vi "data_process_packet.vi"(8 "error in (no error)":errorcluster, 10 "T_offset":u32, 11 "Data Packet":string) -> (0 "error out":errorcluster, 1 "Sensor Packets Returned":i32, 2 "Sensor Readings (Signed)":i16[](array[numeric]), 3 "Time":u32)   [LabVIEW 2018]
panel:
  out "Time Packet":string
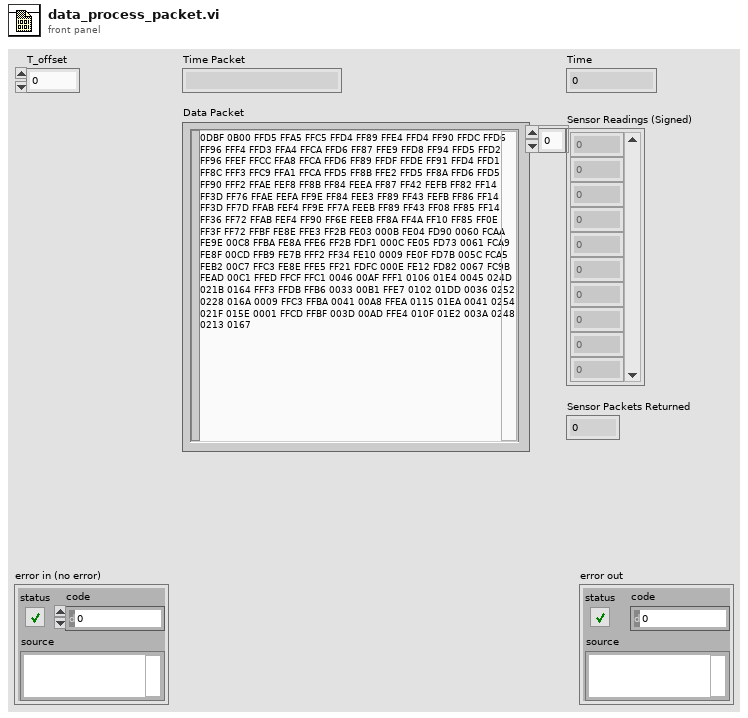
[diagram p1: front panel]
types:
  T1 = enum16{"big-endian, network order", "native, host order", "little-endian"}
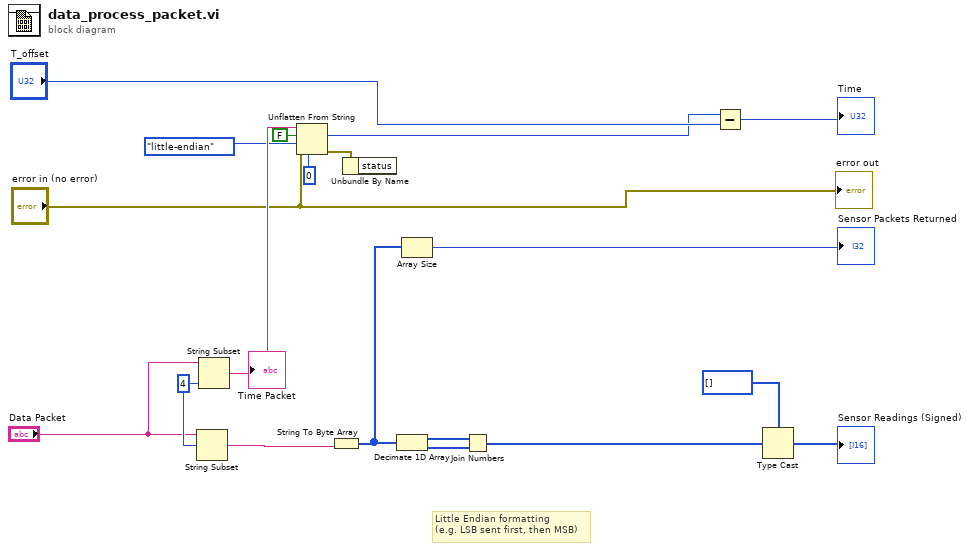
[diagram p0: block diagram]
diagram:
  w19 = 4 ("length (rest)")
  # "Little Endian formatting\n(e.g. LSB sent first, then MSB)"
  n1 = String Subset(string="Data Packet", offset (0)=w19) -> (substring=w16:string)  [unwired: 1 in]
  n2 = String Subset(string="Data Packet", length (rest)=w19) -> (substring=w18:string)  [unwired: 1 in]
  "Time Packet" <- w18
  n3 = Unflatten From String(type=u32 0 ("default (0 U32)"), binary string=w18, data includes array or string size? (T)=FALSE, byte order (0:big-endian, network order)=T1."little-endian", error in (no error)="error in (no error)") -> (value=w2:u32, error out=w4:errorcluster)  [unwired: 1 out]
  n4 = String To Byte Array(string=w16) -> (unsigned byte array=w15:u8[])
  n5 = Unbundle By Name(w4) -> ()  [unwired: 1 out]
  n6 = Decimate 1D Array(w15) -> (w12:u8[], w11:u8[])
  n7 = Array Size(array=w15) -> (size(s)=→"Sensor Packets Returned":i32)
  n8 = Join Numbers(hi=w12, lo=w11) -> ((hi.lo)=w9:u16[])
  n9 = Subtract(x=w2, y="T_offset") -> (x-y=→"Time":u32)
  n10 = Type Cast(type=i16[] [], x=w9) -> (*(type *) &x=→"Sensor Readings (Signed)":i16[])
  "error out" <- "error in (no error)"
